vi "Get Total Result.vi"(8 "error in (no error)":errorcluster, 11 "MCLB_Lib in":refnum<class "MCLB_Lib.lvclass">) -> (0 "error out":errorcluster, 2 "TotalResult T: OK":bool, 3 "MCLB_Lib out":refnum<class "MCLB_Lib.lvclass">)   [LabVIEW 2021, in "MCLB_Lib.lvclass"]
uses:
  <userlib>/John_Lib/MCLB/MCLB_Lib.lvclass
  <userlib>/John_Lib/MCLB/MCLB_Lib.lvclass/MCLB_Lib.ctl
  e7717c27-2bbc-406c-a878-886e9603b3af.vi
  cc070cab-0521-4761-a62b-45da62386173.vi
panel:
  out "Item Names":string[][](array[string])
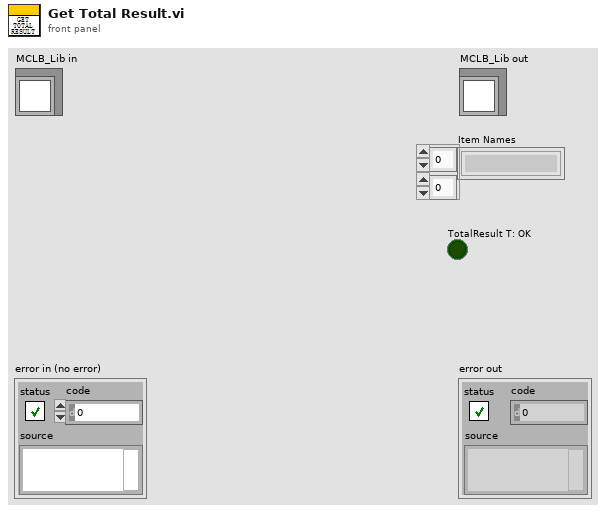
[diagram p1: front panel]
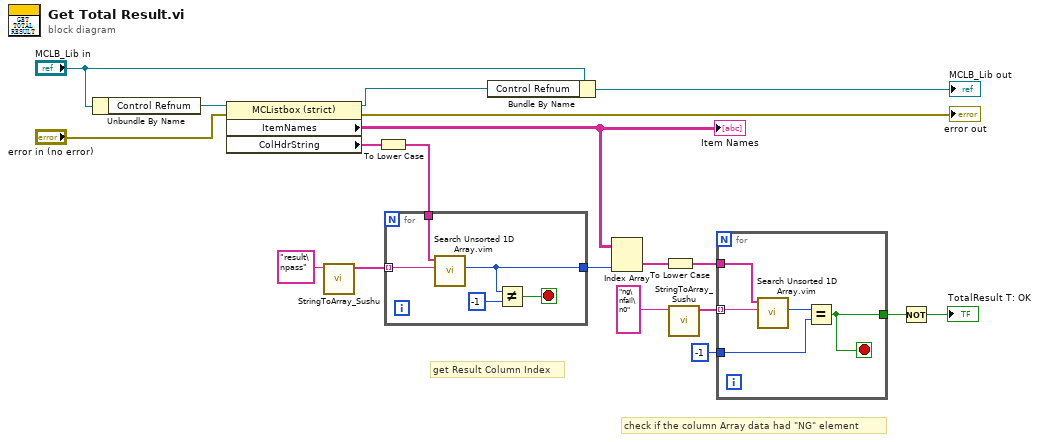
[diagram p0: block diagram]
diagram:
  # "check if the column Array data had \"NG\" element"
  # "get Result Column Index"
  n1 = Unbundle By Name("MCLB_Lib in") -> ("Control Refnum"=w7:refnum<vi>)
  n2 = property class="MCListbox (strict)"(reference=w7, error in="error in (no error)") -> (reference out=w3:refnum<vi>, error out=→"error out":errorcluster, "ItemNames"=w1:string[][], "ColHdrString"=w10:string[])
  "Item Names" <- w1
  n3 = call <userlib>:"StringToArray_Sushu.vi"("State Queue"="result\npass") -> ("Array"=w9:string[])  [unwired: 7 in, 3 out]
  n4 = To Lower Case(string=w10) -> (all lower case string=w11:string[])
  n5 = for {
    tunnel: [w22] -> w5
    tunnel: w11 -> [w24]
    tunnel: w9 -> [w23] mode=indexing
    stop <- w20 stop-if-true
    n6 = call "Search Unsorted 1D Array.vim"("element"=w23, "unsorted 1D array"=w24) -> ("index of element"=w22:i32)  [unwired: 9 in]
    n7 = Not Equal?(x=w22, y=-1) -> (x != y?=w20:bool)
  }
  n8 = Bundle By Name(cluster="MCLB_Lib in", "Control Refnum"=w3) -> (→"MCLB_Lib out":refnum<class "MCLB_Lib.lvclass">)
  n9 = Index Array(array=w1, index (col)=w5) -> (element=w18:string[])  [unwired: 1 in]
  n10 = To Lower Case(string=w18) -> (all lower case string=w16:string[])
  n11 = call <userlib>:"StringToArray_Sushu.vi"("State Queue"="ng\nfail\n0") -> ("Array"=w15:string[])  [unwired: 7 in, 3 out]
  n12 = for {
    tunnel: w16 -> [w26]
    tunnel: w15 -> [w25] mode=indexing
    tunnel: -1 ("y") -> [w28]
    tunnel: [w27] -> w13
    stop <- w27 stop-if-true
    n13 = call "Search Unsorted 1D Array.vim"("element"=w25, "unsorted 1D array"=w26) -> ("index of element"=w29:i32)  [unwired: 9 in]
    n14 = Equal?(x=w29, y=w28) -> (x = y?=w27:bool)
  }
  n15 = Not(x=w13) -> (.not. x?=→"TotalResult T: OK":bool)
